vi "Convert to Interface State.vi"(8 "error in (no error)":errorcluster, 11 "Instrument State in":T2) -> (0 "error out":errorcluster, 3 "Instrument State Out":variant)   [LabVIEW 2020, in "Polar Bear Plus All-in-One Plugin.lvlib" / "Remote Connection Manager.lvlib"]
uses:
  Remote Connection Manager.lvlib
  Instrument Manager/Instrument State.ctl
  <instrlib>/RxnRover/Driver Polar Bear Plus/heater_parent/heater_parent.lvclass
  Typedefs/Remote Temperature Controller State.ctl
  Polar Bear Plus All-in-One Plugin.lvlib
  Instrument Manager/Instrument Manager.lvlib
panel:
  out "Remote Temperature Controller State":T1
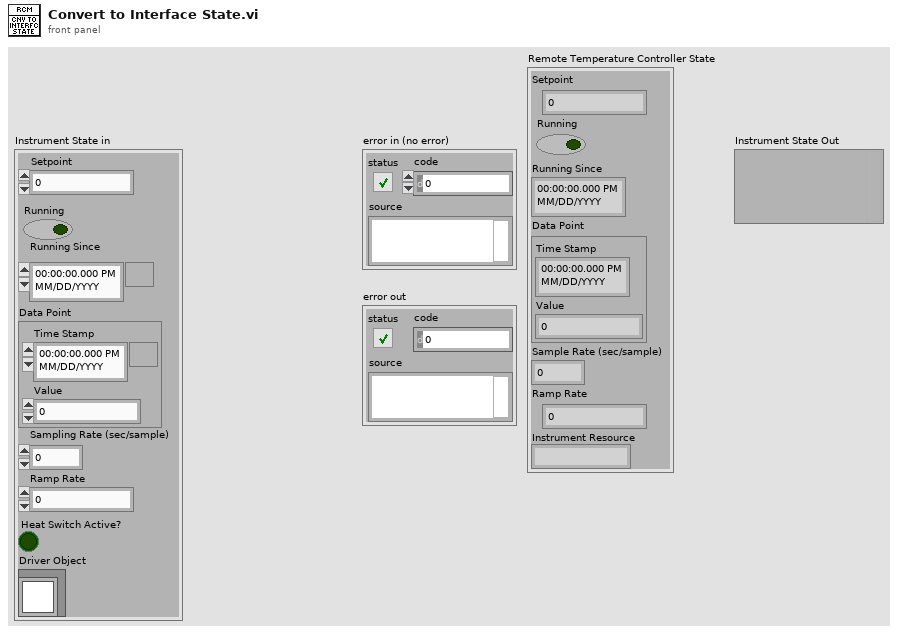
[diagram p1: front panel]
types:
  T1 = typedef "Polar Bear Plus All-in-One Plugin.lvlib/Remote Temperature Controller State.ctl" = cluster{"Setpoint":dbl, "Running":bool, "Running Since":timestamp, "Data Point":cluster{"Time Stamp":timestamp, "Value":dbl}, "Sample Rate (sec/sample)":dbl, "Ramp Rate":dbl, "Instrument Resource":string}
  T2 = typedef "Polar Bear Plus All-in-One Plugin.lvlib/Instrument Manager.lvlib/Instrument State.ctl" = cluster{"Setpoint":dbl, "Running":bool, "Running Since":timestamp, "Data Point":cluster{"Time Stamp":timestamp, "Value":dbl}, "Sampling Rate (sec/sample)":dbl, "Ramp Rate":dbl, "Heat Switch Active?":bool, "Driver Object":refnum<class "heater_parent.lvclass">}
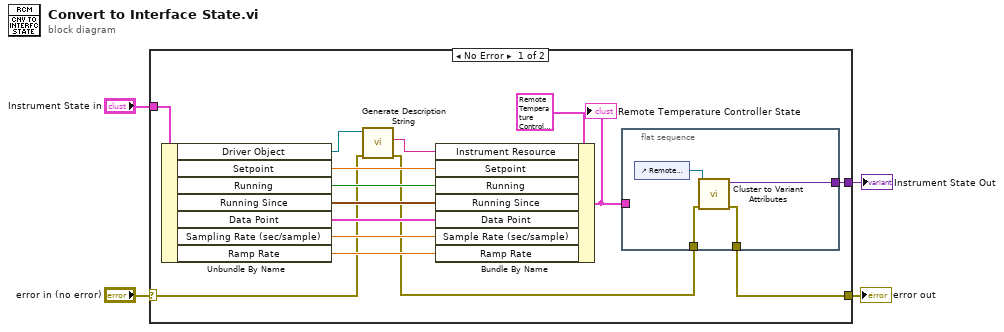
[diagram p0: block diagram]
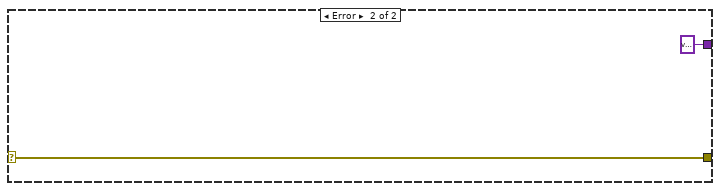
[diagram p2: hidden frame]
diagram:
  n1 = case shown="No Error" "error in (no error)" {
    selector: "error in (no error)" -> [w7 w25]
    tunnel: "Instrument State in" -> [w18 _]
    tunnel: [w12 w25] -> w2
    tunnel: [w10 variant ("Variant out")] -> w1
    frame No Error {
      n2 = Unbundle By Name(w18) -> ("Driver Object"=w8:refnum<class "heater_parent.lvclass">, "Setpoint"=w17:dbl, "Running"=w16:bool, "Running Since"=w15:timestamp, "Data Point"=w14:cluster{"Time Stamp":timestamp, "Value":dbl}, "Sampling Rate (sec/sample)"=w13:dbl, "Ramp Rate"=w9:dbl)
      n3 = call-dynamic "Generate Description String.vi"("error in (no error)"=w7, "heater_parent in"=w8) -> ("error out"=w6:errorcluster, "Description String"=w5:string)  [unwired: 7 in, 1 out]
      n4 = Bundle By Name(cluster=T1 {"Setpoint"=0.0, "Running"=FALSE, "Running Since"=timestamp(0 s since 1904-01-01), "Data Point"={"Time Stamp"=timestamp(0 s since 1904-01-01), "Value"=0.0}, "Sample Rate (sec/sample)"=0.0, "Ramp Rate"=0.0, "Instrument Resource"=""} ("Instrument State"), "Instrument Resource"=w5, "Setpoint"=w17, "Running"=w16, "Running Since"=w15, "Data Point"=w14, "Sample Rate (sec/sample)"=w13, "Ramp Rate"=w9) -> (w11:T1)
      "Remote Temperature Controller State" <- w11
      n5 = flat-sequence {
        tunnel: w6 -> [w23]
        tunnel: [w22] -> w12
        tunnel: w11 -> [_]
        tunnel: [w20] -> w10
        frame #0 {
          n6 = control-ref of="Remote Temperature Controller State"() -> (w21:refnum<vi>)
          n7 = call "Cluster to Variant Attributes.vi"("error in (no error)"=w23, "Cluster in"=w21) -> ("error out"=w22:errorcluster, "Variant out"=w20:variant)  [unwired: 8 in]
        }
      }
    }
    frame Error {
    }
  }
  "error out" <- w2
  "Instrument State Out" <- w1
